vi "Calculate trigger period.vi"(4 "Tadj [us]":dbl=0.4, 6 "Ny":u16, 9 "AOD Fill":dbl, 10 "Tdwell [us]":dbl, 11 "Nx":u16) -> (3 "period":u32)   [LabVIEW 2020]
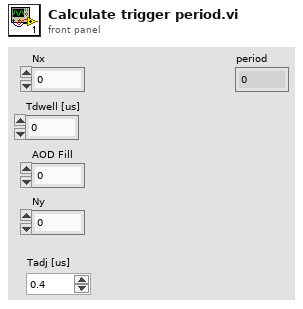
[diagram p1: front panel]
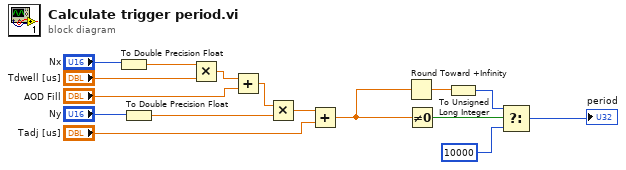
[diagram p0: block diagram]
diagram:
  n1 = To Double Precision Float(number="Nx") -> (double precision float=w9:dbl)
  n2 = To Double Precision Float(number="Ny") -> (double precision float=w7:dbl)
  n3 = Multiply(x=w9, y="Tdwell [us]") -> (x*y=w14:dbl)
  n4 = Add(x=w14, y="AOD Fill") -> (x+y=w12:dbl)
  n5 = Multiply(x=w12, y=w7) -> (x*y=w3:dbl)
  n6 = Add(x=w3, y="Tadj [us]") -> (x+y=w1:dbl)
  n7 = Round Toward +Infinity(x=w1) -> (ceil(x): smallest int >= x=w4:dbl)
  n8 = Not Equal To 0?(x=w1) -> (x != 0?=w11:bool)
  n9 = To Unsigned Long Integer(number=w4) -> (unsigned 32bit integer=w6:u32)
  n10 = Select(t=w6, s=w11, f=u32 10000) -> (s? t:f=→"period":u32)
